vi "Convolution.vi"   [LabVIEW 2020, in "NI_AALPro.lvlib"]
doc: "Computes the convolution of the input sequences <B>X</B> and <B>Y</B>. Wire data to the <B>X</B> and <B>Y</B> inputs to determine the polymorphic instance to use or manually select the instance."
uses:
  <vilib>/Analysis/NI_AALPro.lvlib
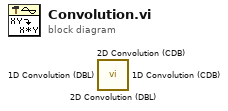
[diagram p0: block diagram]
diagram:
  n1 = call <vilib>:"2D Convolution (DBL).vi"() -> ()  [unwired: 10 in, 2 out]
  n2 = call <vilib>:"2D Convolution (CDB).vi"() -> ()  [unwired: 10 in, 2 out]
  n3 = call <vilib>:"1D Convolution (DBL).vi"() -> ()  [unwired: 10 in, 2 out]
  n4 = call <vilib>:"1D Convolution (CDB).vi"() -> ()  [unwired: 10 in, 2 out]
